vi "Write Sharpness.vi"(8 "error in":errorcluster, 10 "Sharpness":dbl, 11 "Camera in":refnum<class "Camera.lvclass">) -> (0 "error out":errorcluster, 3 "Camera out":refnum<class "Camera.lvclass">)   [LabVIEW 2018, in "Camera.lvlib" / "Camera.lvclass"]
uses:
  Camera.lvclass
  Camera.lvclass/Camera.ctl
  Custom Controls/Camera Setting.ctl
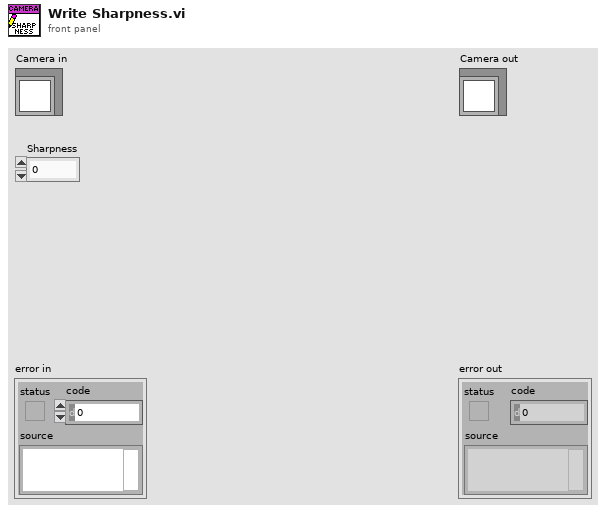
[diagram p1: front panel]
types:
  T1 = typedef "Camera.lvlib/Camera.lvclass/Camera Setting.ctl" = enum16{"Brightness", "Rotation", "Contrast", "Exposure", "Frame Rate", "Gain", "Gamma", "Image Resolution", "Sharpness"}
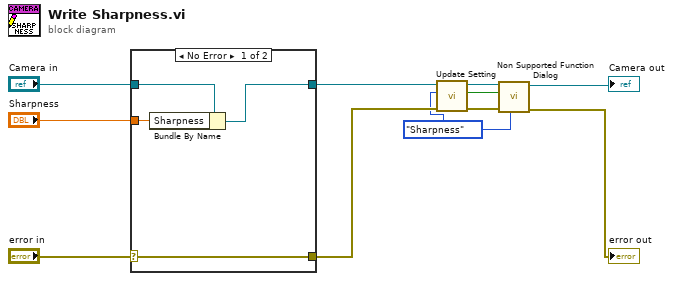
[diagram p0: block diagram]
diagram:
  w1 = Camera_Setting."Sharpness" ("Update Setting:")
  n1 = case shown="No Error" "error in" {
    selector: "error in" -> [w15 w16]
    tunnel: [w15 w16] -> w7
    tunnel: [w13 w17] -> w8
    tunnel: "Camera in" -> [w14 w17]
    tunnel: "Sharpness" -> [w12 _]
    frame No Error {
      n2 = Bundle By Name(cluster=w14, "Sharpness"=w12) -> (w13:refnum<class "Camera.lvclass">)
    }
    frame Error {
    }
  }
  n3 = call-dynamic "Update Setting.vi"("Camera in"=w8, "Setting"=w1, "error in"=w7) -> ("Camera out"=w4:refnum<class "Camera.lvclass">, "Supported?"=w5:bool, "error out"=w6:errorcluster)  [unwired: 5 in]
  n4 = call "Non Supported Function Dialog.vi"("Update Setting:"=w1, "error in"=w6, "Supported?"=w5, "Camera in"=w4) -> ("error out"=→"error out":errorcluster, "Camera out"=→"Camera out":refnum<class "Camera.lvclass">)  [unwired: 6 in]
